vi "New.vi"(8 "error in (no error)":errorcluster, 11 "reference in":refnum<class "Nested Endpoint Test Suite.lvclass">) -> (0 "error out":errorcluster, 3 "reference out":refnum<class "Nested Endpoint Test Suite.lvclass">)   [LabVIEW 2015, in "Nested Endpoint Test Suite.lvclass"]
uses:
  Nested Endpoint Test Suite.lvclass
  Test Network Stream Disconnect/Test Network Stream Disconnect.lvclass
  Test Network Stream Initiator Connect/Test Network Stream Initiator Connect.lvclass
  Test Network Stream Listener Connect/Test Network Stream Listener Connect.lvclass
  Test Network Stream Transmission/Test Network Stream Transmission.lvclass
  Test Network Stream Nested Endpoint/Test Network Stream Nested Endpoint.lvclass
  Test TCP Nested Endpoint/Test TCP Nested Endpoint.lvclass
  Test TCP Nested Endpoint Nonforwarded Messages/Test TCP Nested Endpoint Nonforwarded Messages.lvclass
  Test TCP Stream Disconnect/Test TCP Stream Disconnect.lvclass
  Test TCP Stream Initiator Connect/Test TCP Stream Initiator Connect.lvclass
  Test TCP Stream Listener Connect/Test TCP Stream Listener Connect.lvclass
  Test TCP Stream Transmission/Test TCP Stream Transmission.lvclass
  Test Data Stream/Test Data Stream.lvclass
  <vilib>/addons/_JKI Toolkits/VI Tester/TestCase.llb/TestCase.lvclass
  Nested Endpoint Test Suite.lvclass/Nested Endpoint Test Suite.ctl
  <vilib>/addons/_JKI Toolkits/VI Tester/TestSuite.llb/TestSuite.lvclass
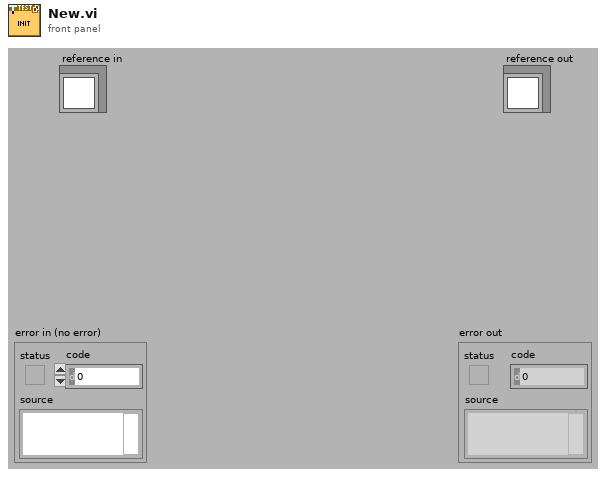
[diagram p1: front panel]
types:
  T1 = cluster{"Test Network Stream Disconnect.lvclass":refnum<class "Test Network Stream Disconnect.lvclass">, "Test Network Stream Initiator Connect.lvclass":refnum<class "Test Network Stream Initiator Connect.lvclass">, "Test Network Stream Listener Connect.lvclass":refnum<class "Test Network Stream Listener Connect.lvclass">, "Test Network Stream Transmission.lvclass":refnum<class "Test Network Stream Transmission.lvclass">, "Test Network Stream Nested Endpoint.lvclass":refnum<class "Test Network Stream Nested Endpoint.lvclass">, "Test TCP Nested Endpoint.lvclass":refnum<class "Test TCP Nested Endpoint.lvclass">, "Test TCP Nested Endpoint Nonforwarded Messages.lvclass":refnum<class "Test TCP Nested Endpoint Nonforwarded Messages.lvclass">, "Test TCP Stream Disconnect.lvclass":refnum<class "Test TCP Stream Disconnect.lvclass">, "Test TCP Stream Initiator Connect.lvclass":refnum<class "Test TCP Stream Initiator Connect.lvclass">, "Test TCP Stream Listener Connect.lvclass":refnum<class "Test TCP Stream Listener Connect.lvclass">, "Test TCP Stream Transmission.lvclass":refnum<class "Test TCP Stream Transmission.lvclass">, "Test Data Stream.lvclass":refnum<class "Test Data Stream.lvclass">}
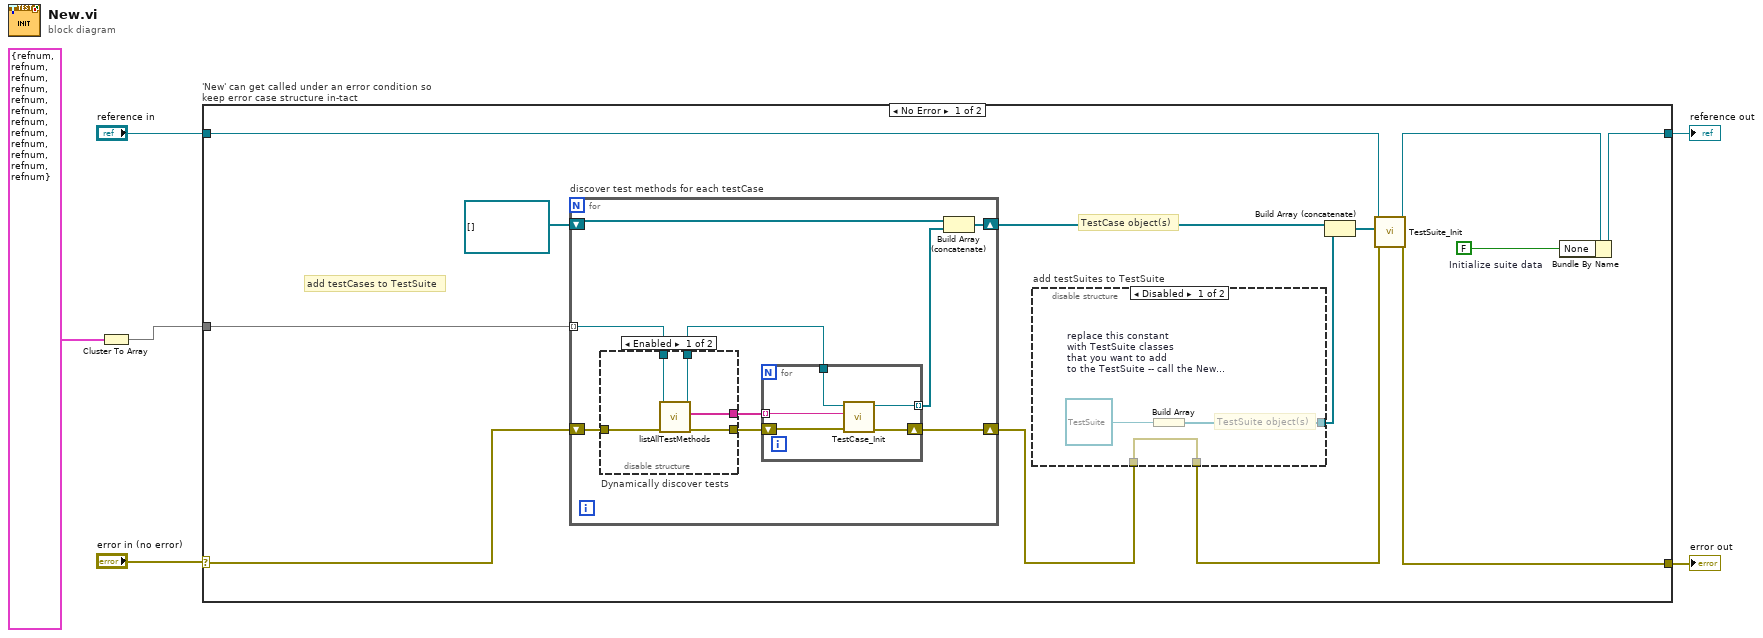
[diagram p0: block diagram]
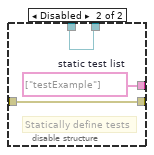
[diagram p2: hidden frame]
diagram:
  n1 = Cluster To Array(cluster=T1 {"Test Network Stream Disconnect.lvclass"=refnum, "Test Network Stream Initiator Connect.lvclass"=refnum, "Test Network Stream Listener Connect.lvclass"=refnum, "Test Network Stream Transmission.lvclass"=refnum, "Test Network Stream Nested Endpoint.lvclass"=refnum, "Test TCP Nested Endpoint.lvclass"=refnum, "Test TCP Nested Endpoint Nonforwarded Messages.lvclass"=refnum, "Test TCP Stream Disconnect.lvclass"=refnum, "Test TCP Stream Initiator Connect.lvclass"=refnum, "Test TCP Stream Listener Connect.lvclass"=refnum, "Test TCP Stream Transmission.lvclass"=refnum, "Test Data Stream.lvclass"=refnum}) -> (array=w1:refnum<class "TestCase.lvclass">[])
  n2 = case "'New' can get called under an error condition so keep error case structure in-tact" shown="No Error" "error in (no error)" {
    selector: "error in (no error)" -> [w14 w46]
    tunnel: [w19 w47] -> w6
    tunnel: "reference in" -> [w15 w47]
    tunnel: [w16 w46] -> w3
    tunnel: w1 -> [w7 _]
    frame No Error {
      w18 = FALSE  # Initialize suite data
      # "TestCase object(s)"
      # "add testCases to TestSuite"
      n3 = for "discover test methods for each testCase" {
        shift-right: [w28] -> w9
        shift-left: w14 -> [w24]
        tunnel: w7 -> [w21] mode=indexing
        shift-right: [w25] -> w13
        shift-left: refnum<class "TestCase.lvclass">[] [] -> [w26]
        n4 = disable-structure "Dynamically discover tests" shown="Enabled" {
          disable-tunnel: w24 -> [w33 w34]
          disable-tunnel: [w32 w34] -> w23
          disable-tunnel: [w31 w35] -> w22
          disable-tunnel: w21 -> [w30 w36]
          disable-tunnel: [w29 w36] -> w20
          frame Enabled {
            n5 = call-dynamic "listAllTestMethods.vi"("error in (no error)"=w33, "TestCase in"=w30) -> ("error out"=w32:errorcluster, "test methods"=w31:string[], "TestCase out"=w29:refnum<class "TestCase.lvclass">)  [unwired: 7 in]
          }
          frame Disabled {
            w35 = string[] ["testExample"]  # static test list
            # "Statically define tests"
          }
        }
        n6 = for {
          tunnel: w20 -> [w37]
          tunnel: w22 -> [w41] mode=indexing
          shift-right: [w39] -> w28
          shift-left: w23 -> [w40]
          tunnel: [w38] -> w27 mode=indexing
          n7 = call <vilib>:"TestCase_Init.vi"("error in (no error)"=w40, "methodName (\"runTest\")"=w41, "TestCase in"=w37) -> ("error out"=w39:errorcluster, "TestCase out"=w38:refnum<class "TestCase.lvclass">)  [unwired: 7 in]
        }
        n8 = Build Array (concatenate)(w26, w27) -> (w25:refnum<class "TestCase.lvclass">[])
      }
      n9 = disable-structure "add testSuites to TestSuite" shown="Disabled" {
        disable-tunnel: [w42 _] -> w11
        disable-tunnel: [w44 w45] -> w10
        disable-tunnel: w9 -> [w44 w45]
        frame Disabled {
          w43 = refnum<class "TestSuite.lvclass"> refnum  # replace this constant with TestSuite classes that you want to add to the TestSuite -- call the New method for each TestSuite prior to adding it to this TestSuite
          # "TestSuite object(s)"
          n10 = Build Array(w43) -> (w42:refnum<class "TestSuite.lvclass">[])
        }
        frame Enabled {
          # "by default, no TestSuites are defined\nas members of a TestSuite"
        }
      }
      n11 = Build Array (concatenate)(w13, w11) -> (w12:refnum<class>[])
      n12 = call <vilib>:"TestSuite_Init.vi"("error in (no error)"=w10, "tests (none)"=w12, "TestSuite in"=w15) -> ("error out"=w16:errorcluster, "TestSuite out"=w17:refnum<class "Nested Endpoint Test Suite.lvclass">)  [unwired: 7 in]
      n13 = Bundle By Name(cluster=w17, "None"=w18) -> (w19:refnum<class "Nested Endpoint Test Suite.lvclass">)
    }
    frame Error {
    }
  }
  "reference out" <- w6
  "error out" <- w3
